vi "process_layer_parameter_strict_type_to_strings.vi"(8 "error in (no error)":errorcluster, 10 "Process layer parameters":T1) -> (0 "error out":errorcluster, 2 "Process layer parameters (strings)":T2)   [LabVIEW 2018]
uses:
  process_layer_parameters_strings.ctl
  process_layer_parameters.ctl
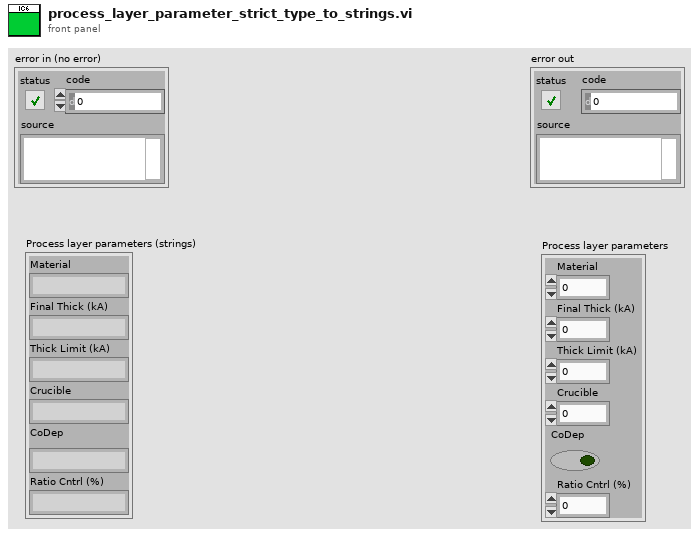
[diagram p1: front panel]
types:
  T1 = typedef "process_layer_parameters.ctl" = cluster{"Material":u8, "Final Thick (kA)":sgl, "Thick Limit (kA)":sgl, "Crucible":u8, "CoDep":bool, "Ratio Cntrl (%)":sgl}
  T2 = typedef "process_layer_parameters_strings.ctl" = cluster{"Material":string, "Final Thick (kA)":string, "Thick Limit (kA)":string, "Crucible":string, "CoDep":string, "Ratio Cntrl (%)":string}
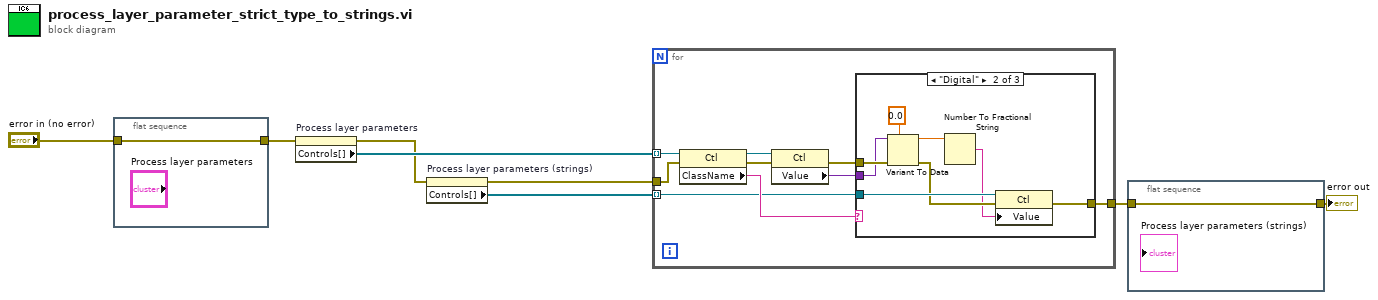
[diagram p0: block diagram]
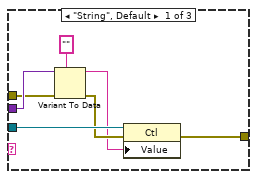
[diagram p2: hidden frame]
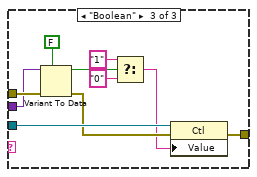
[diagram p3: hidden frame]
diagram:
  n1 = flat-sequence {
    tunnel: "error in (no error)" -> [w9]
    tunnel: [w9] -> w3
    frame #0 {
    }
  }
  n2 = property on="Process layer parameters" class="Clust (strict)"(error in=w3) -> (error out=w1:errorcluster, "Controls[]"=w2:refnum<vi>[])  [unwired: 1 in, 1 out]
  n3 = property on="Process layer parameters (strings)" class="Clust (strict)"(error in=w1) -> (error out=w5:errorcluster, "Controls[]"=w4:refnum<vi>[])  [unwired: 1 in, 1 out]
  n4 = for {
    tunnel: w2 -> [w12] mode=indexing
    tunnel: w4 -> [w10] mode=indexing
    tunnel: w5 -> [w11]
    tunnel: [w18] -> w7
    n5 = property class="Ctl"(reference=w12, error in=w11) -> (reference out=w13:refnum<vi>, error out=w14:errorcluster, "ClassName"=w15:string)
    n6 = property class="Ctl"(reference=w13, error in=w14) -> (error out=w17:errorcluster, "Value"=w16:variant)  [unwired: 1 out]
    n7 = case shown="\"Digital\"" w15 {
      tunnel: w10 -> [w24 w33 w43]
      tunnel: [w25 w32 w42] -> w18
      tunnel: w17 -> [w22 w30 w41]
      tunnel: w16 -> [w23 w29 w40]
      frame "String", Default {
        n8 = Variant To Data(error in=w22, type="", Variant=w23) -> (data=w19:string, error out=w20:errorcluster)
        n9 = property class="Ctl"(reference=w24, error in=w20, "Value"=w19) -> (error out=w25:errorcluster)  [unwired: 1 out]
      }
      frame "Digital" {
        n10 = Variant To Data(error in=w30, type=0.0, Variant=w29) -> (data=w27:dbl, error out=w28:errorcluster)
        n11 = Number To Fractional String(number=w27) -> (F-format string=w26:string)  [unwired: 3 in]
        n12 = property class="Ctl"(reference=w33, error in=w28, "Value"=w26) -> (error out=w32:errorcluster)  [unwired: 1 out]
      }
      frame "Boolean" {
        n13 = Variant To Data(error in=w41, type=FALSE, Variant=w40) -> (data=w37:bool, error out=w39:errorcluster)
        n14 = Select(t="1", s=w37, f="0") -> (s? t:f=w34:string)
        n15 = property class="Ctl"(reference=w43, error in=w39, "Value"=w34) -> (error out=w42:errorcluster)  [unwired: 1 out]
      }
    }
  }
  n16 = flat-sequence {
    tunnel: w7 -> [w44]
    tunnel: [w44] -> w6
    frame #0 {
    }
  }
  "error out" <- w6
